vi "MMI_AC_StrDismantle.vi"(1 "LogEvent":refnum<vi>, 2 "VCI_CAN_OBJ_R":T1) -> (0 "MMI_AC_CmdCluster":T2 {"空气质量弹窗提醒" items=["未按下", "取消提醒"]; "驻车空调设置" items=["无", "关闭", "开启"]; "左侧设定温度" scale=17.5..31.5; "吹风模式请求" items=["Face", "Bilevel", "Foot", "Foot Screen", "Screen", "未设置"]; "鼓风机风速档位" items=["关闭", "风速1", "风速2", "风速3", "风速4", "风速5", "风速6", "风速7", "风速8", "未设置"]})   [LabVIEW 2013]
uses:
  Log.ctl
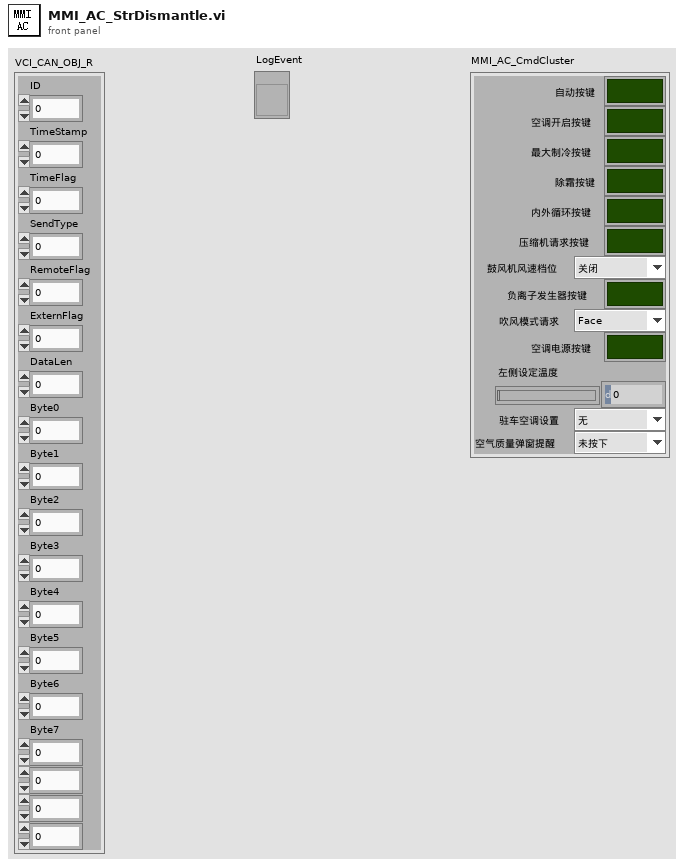
[diagram p1: front panel]
types:
  T1 = cluster{"ID":u32, "TimeStamp":u32, "TimeFlag":u8, "SendType":u8, "RemoteFlag":u8, "ExternFlag":u8, "DataLen":u8, "Byte0":u8, "Byte1":u8, "Byte2":u8, "Byte3":u8, "Byte4":u8, "Byte5":u8, "Byte6":u8, "Byte7":u8, u8, u8, u8}
  T2 = cluster{"自动按键":bool, "空调开启按键":bool, "最大制冷按键":bool, "除霜按键":bool, "内外循环按键":bool, "压缩机请求按键":bool, "鼓风机风速档位":u16, "负离子发生器按键":bool, "吹风模式请求":u16, "空调电源按键":bool, "左侧设定温度":dbl, "驻车空调设置":u16, "空气质量弹窗提醒":u16}
  T3 = typedef "Log.ctl" = cluster{"Event":string, "Value":variant}
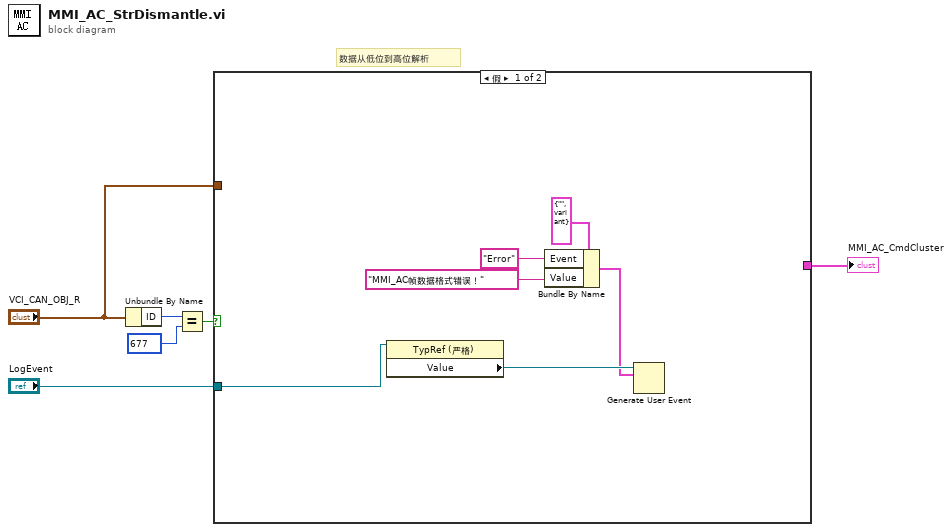
[diagram p0: block diagram]
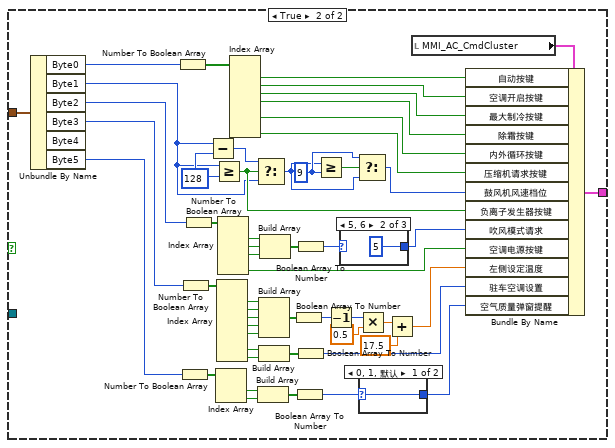
[diagram p2: hidden frame]
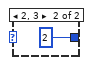
[diagram p3: hidden frame]
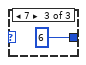
[diagram p5: hidden frame]
diagram:
  # "数据从低位到高位解析"
  n1 = Unbundle By Name("VCI_CAN_OBJ_R") -> ("ID"=w5:u32)
  n2 = Equal?(x=w5, y=u16 677) -> (x = y?=w3:bool)
  n3 = case shown="假" w3 {
    tunnel: [_ w42] -> w6
    tunnel: "VCI_CAN_OBJ_R" -> [_ w18]
    tunnel: "LogEvent" -> [w7 _]
    frame False {
      n4 = property class="TypRef (严格)"(reference=w7) -> ("Value"=w12:refnum<user-event>)  [unwired: 1 in, 2 out]
      n5 = Bundle By Name(cluster=T3 {"Event"="", "Value"=variant} ("Log"), "Event"="Error", "Value"="MMI_AC帧数据格式错误！" ("消息")) -> (w9:T3)
      n6 = Generate User Event(user event=w12, event data cluster=w9) -> ()  [unwired: 2 in, 2 out]
    }
    frame True {
      w53 = u8 128 ("y")
      w56 = u8 9 ("y")
      n7 = Unbundle By Name(w18) -> ("Byte0"=w17:u8, "Byte1"=w16:u8, "Byte2"=w15:u8, "Byte3"=w14:u8, "Byte5"=w13:u8)  [unwired: 1 out]
      n8 = Number To Boolean Array(number=w17) -> (Boolean array=w64:bool[])
      n9 = Number To Boolean Array(number=w13) -> (Boolean array=w24:bool[])
      n10 = Number To Boolean Array(number=w14) -> (Boolean array=w41:bool[])
      n11 = Number To Boolean Array(number=w15) -> (Boolean array=w50:bool[])
      n12 = Subtract(x=w16, y=w53) -> (x-y=w54:u8)
      n13 = Greater Or Equal?(x=w16, y=w53) -> (x >= y?=w52:bool)
      n14 = Index Array(array=w24) -> (element #1=w21:bool, element #2=w22:bool)  [unwired: 2 in]
      n15 = Index Array(array=w41) -> (element #1=w40:bool, element #2=w39:bool, element #3=w38:bool, element #4=w37:bool, element #5=w36:bool, element #7=w28:bool, element #8=w27:bool)  [unwired: 8 in, 1 out]
      n16 = Index Array(array=w50) -> (element #1=w49:bool, element #2=w48:bool, element #3=w47:bool, element #5=w45:bool)  [unwired: 5 in, 1 out]
      n17 = Index Array(array=w64) -> (element #1=w63:bool, element #2=w62:bool, element #3=w61:bool, element #4=w60:bool, element #6=w59:bool, element #8=w58:bool)  [unwired: 8 in, 2 out]
      n18 = Select(t=w54, s=w52, f=w16) -> (s? t:f=w51:u8)
      n19 = Build Array(w21, w22) -> (w23:bool[])
      n20 = Build Array(w40, w39, w38, w37, w36) -> (w35:bool[])
      n21 = Build Array(w28, w27) -> (w26:bool[])
      n22 = Build Array(w49, w48, w47) -> (w46:bool[])
      n23 = Boolean Array To Number(Boolean array=w35) -> (number=w34:u32)
      n24 = Boolean Array To Number(Boolean array=w23) -> (number=w20:u32)
      n25 = Boolean Array To Number(Boolean array=w46) -> (number=w44:u32)
      n26 = Boolean Array To Number(Boolean array=w26) -> (number=w25:u32)
      n27 = Greater Or Equal?(x=w51, y=w56) -> (x >= y?=w57:bool)
      n28 = Decrement(x=w34) -> (x-1=w33:u32)
      n29 = case shown="5, 6" w44 {
        selector: w44 -> [w68 _ _]
        tunnel: [w68 5 6] -> w43
        frame 0..4, Default {
        }
        frame 5, 6 {
        }
        frame 7 {
        }
      }
      n30 = Select(t=w56, s=w57, f=w51) -> (s? t:f=w55:u8)
      n31 = Multiply(x=w33, y=0.5) -> (x*y=w31:dbl)
      n32 = case shown="0, 1, 默认" w20 {
        selector: w20 -> [w66 _]
        tunnel: [w66 2] -> w19
        frame 0, 1, Default {
        }
        frame 2, 3 {
        }
      }
      n33 = Add(x=w31, y=17.5) -> (x+y=w29:dbl)
      n34 = local read "MMI_AC_CmdCluster"() -> (w65:T2)
      n35 = Bundle By Name(cluster=w65, "自动按键"=w63, "空调开启按键"=w62, "最大制冷按键"=w61, "除霜按键"=w60, "内外循环按键"=w59, "压缩机请求按键"=w58, "鼓风机风速档位"=w55, "负离子发生器按键"=w52, "吹风模式请求"=w43, "空调电源按键"=w45, "左侧设定温度"=w29, "驻车空调设置"=w25, "空气质量弹窗提醒"=w19) -> (w42:T2)
    }
  }
  "MMI_AC_CmdCluster" <- w6
